vi "Remote Command Sender ver1.vi"() -> ()   [LabVIEW 2016]
panel:
  in  "Max Vacuum":dbl=600.0
  in  "Go 2 Assign Point":bool
  in  "Assign Point":dbl[](array[numeric])=[0.0, 5.0] min=0.5 max=1.5 step=0.05
  out "remote sender engaged":bool
  in  "emergency alarm bit":bool
  in  "Scaling Array":dbl[](array[numeric])=[1.0, 1.0, 1.0] min=0.5 max=1.5 step=0.05
  in  "Rotation Array":dbl[](array[numeric])=[0.0, 0.0, 0.0] min=-30.0 max=30.0 step=1.0
  in  "Translation Array":dbl[](array[numeric])=[0.0, 0.0, 0.0] min=-3.0 max=3.0 step=0.01
  in  "OCT Z-Axis cmd":dbl step=0.5
  in  "stop":bool
  in  "L1":sgl
  in  "L2":sgl
  in  "L3 (L3=20 is RCM)":sgl
  in  "L4":sgl
  in  "gripper":sgl
  in  "down_pedal":sgl format="%.2f"
  in  "up_pedal":bool
  in  "left_pedal":bool
  in  "right_pedal":bool
  in  "StagePosition - X":dbl=6.0
  in  "StagePosition - Y":dbl=6.0
  in  "StagePosition - Z":dbl=6.0
  # "x scaling"
  # "y scaling"
  # "z scaling"
  # "x rotation"
  # "[deg]"
  # "y rotation"
  # "[deg]"
  # "z rotation"
  # "[deg]"
  # "x translation"
  # "[mm]"
  # "y translation"
  # "[mm]"
  # "z translation"
  # "[mm]"
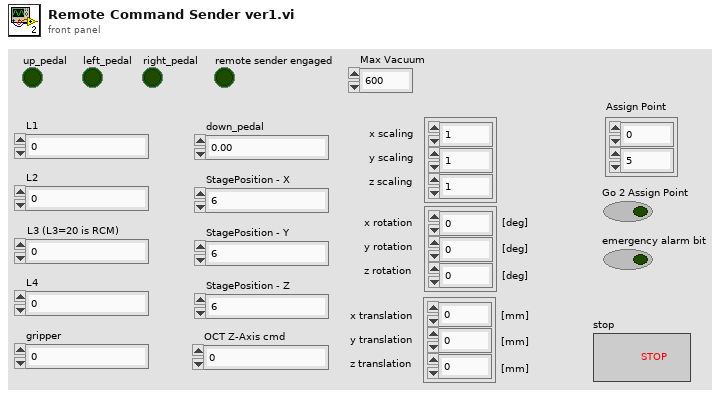
[diagram p1: front panel]
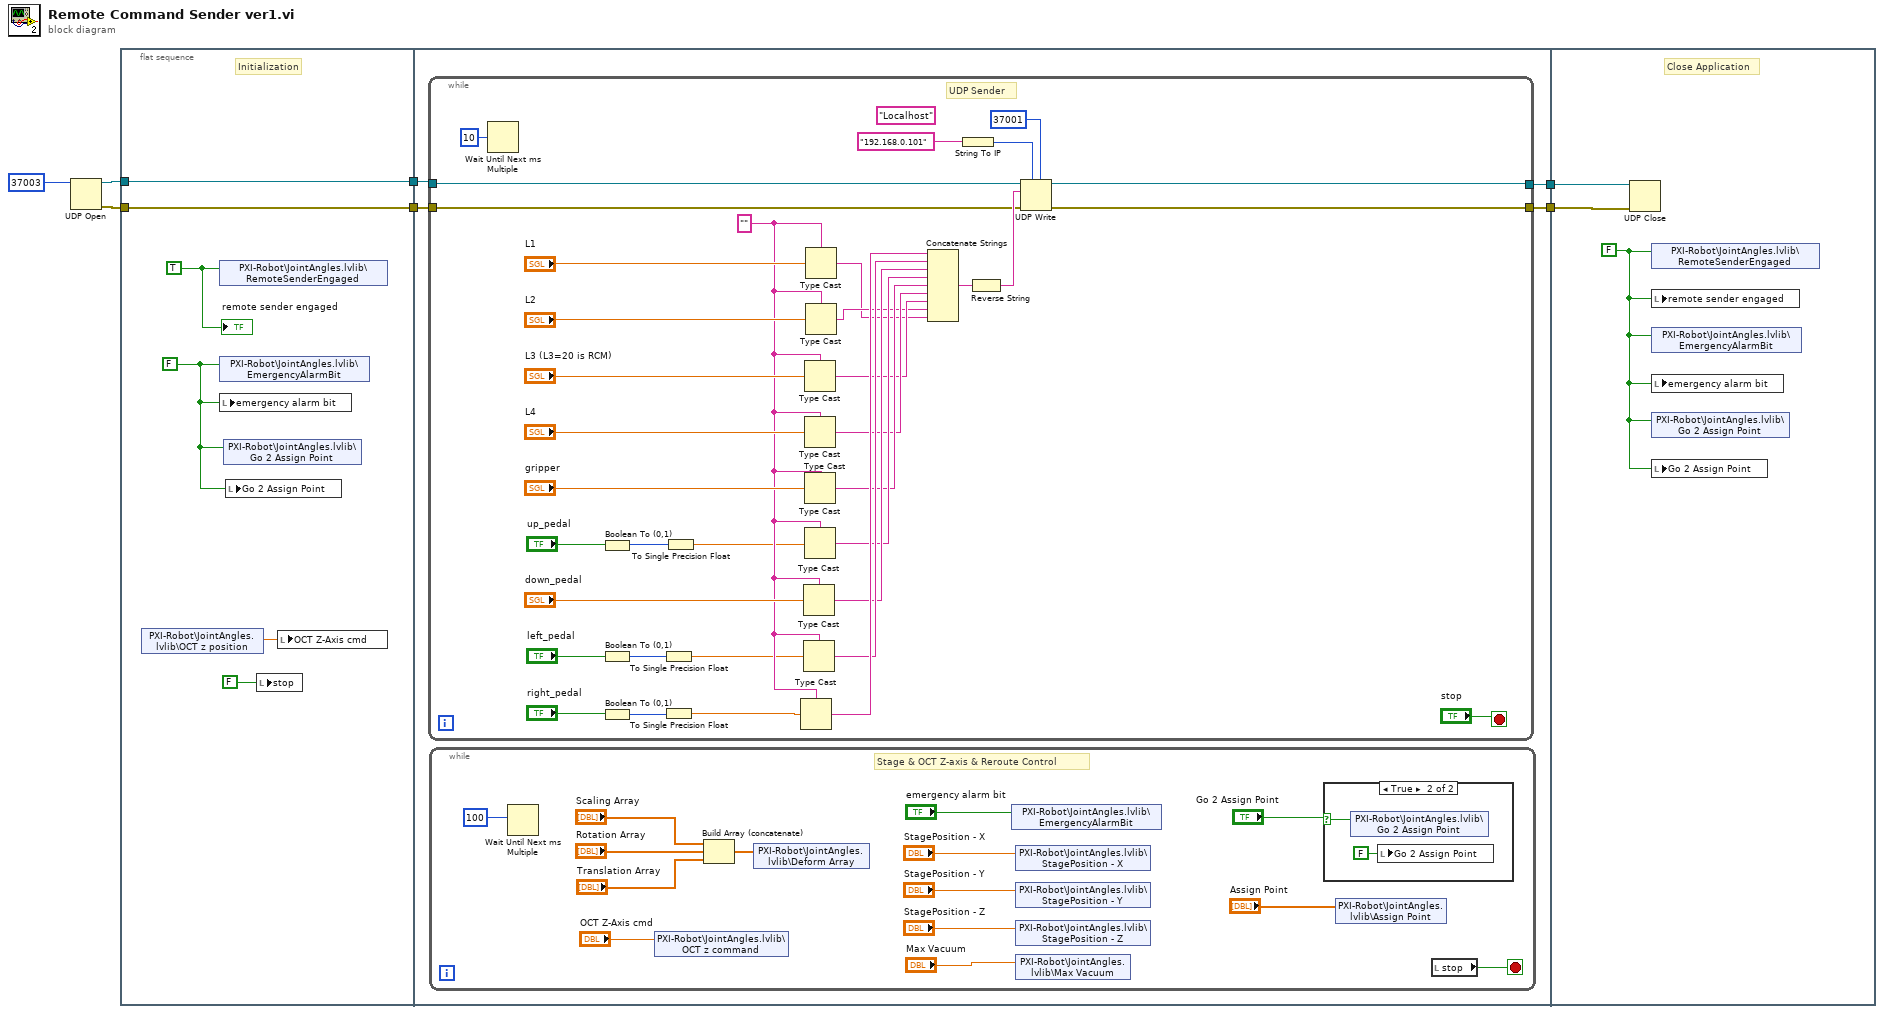
[diagram p0: block diagram]
diagram:
  n1 = UDP Open(11:u16 37003 ("port")) -> (port=w6:refnum<k16>, 0:w5:errorcluster)  [unwired: 4 in, 1 out]
  n2 = flat-sequence {
    tunnel: w5 -> [w12]
    tunnel: w6 -> [w13]
    tunnel: [w13] -> w4
    tunnel: [w12] -> w3
    tunnel: w4 -> [w17]
    tunnel: w3 -> [w16]
    tunnel: [w15] -> w2
    tunnel: [w14] -> w1
    tunnel: w2 -> [w72]
    tunnel: w1 -> [w71]
    frame #0 {
      w8 = FALSE ("EmergencyAlarmBit")
      w10 = TRUE ("RemoteSenderEngaged")
      # "Initialization"
      n3 = shared-variable "PXI-Robot\\JointAngles.lvlib\\OCT z position"() -> (w11:dbl)  [unwired: 1 in, 1 out]
      n4 = shared-variable "PXI-Robot\\JointAngles.lvlib\\RemoteSenderEngaged"(w10) -> ()  [unwired: 1 in, 1 out]
      n5 = shared-variable "PXI-Robot\\JointAngles.lvlib\\EmergencyAlarmBit"(w8) -> ()  [unwired: 1 in, 1 out]
      n6 = local write "emergency alarm bit"(w8) -> ()
      n7 = shared-variable "PXI-Robot\\JointAngles.lvlib\\Go 2 Assign Point"(w8) -> ()  [unwired: 1 in, 1 out]
      n8 = local write "Go 2 Assign Point"(w8) -> ()
      n9 = local write "stop"(FALSE ("stop")) -> ()
      n10 = local write "OCT Z-Axis cmd"(w11) -> ()
      "remote sender engaged" <- w10
    }
    frame #1 {
      n11 = while {
        tunnel: w17 -> [w62]
        tunnel: [w68] -> w15
        tunnel: w16 -> [w61]
        tunnel: [w67] -> w14
        stop <- "stop" stop-if-true
        (unwired) "Localhost" ("reversed")
        w51 = "" ("reversed")
        # "UDP Sender"
        n12 = Wait Until Next ms Multiple(millisecond multiple=u32 10) -> ()  [unwired: 1 out]
        n13 = Boolean To (0,1)(Boolean="up_pedal") -> (0, 1=w41:i16)
        n14 = Boolean To (0,1)(Boolean="left_pedal") -> (0, 1=w37:i16)
        n15 = Boolean To (0,1)(Boolean="right_pedal") -> (0, 1=w39:i16)
        n16 = To Single Precision Float(number=w37) -> (single precision float=w36:sgl)
        n17 = To Single Precision Float(number=w39) -> (single precision float=w38:sgl)
        n18 = To Single Precision Float(number=w41) -> (single precision float=w40:sgl)
        n19 = Type Cast(type=w51, x=w38) -> (*(type *) &x=w50:string)
        n20 = Type Cast(type=w51, x="down_pedal") -> (*(type *) &x=w48:string)
        n21 = Type Cast(type=w51, x=w36) -> (*(type *) &x=w49:string)
        n22 = Type Cast(type=w51, x="L3 (L3=20 is RCM)") -> (*(type *) &x=w44:string)
        n23 = Type Cast(type=w51, x="L4") -> (*(type *) &x=w45:string)
        n24 = Type Cast(type=w51, x="gripper") -> (*(type *) &x=w46:string)
        n25 = Type Cast(type=w51, x=w40) -> (*(type *) &x=w47:string)
        n26 = Type Cast(type=w51, x="L1") -> (*(type *) &x=w42:string)
        n27 = Type Cast(type=w51, x="L2") -> (*(type *) &x=w43:string)
        n28 = Concatenate Strings(w50, w49, w48, w47, w46, w45, w44, w43, w42) -> (w66:string)
        n29 = String To IP(1:"192.168.0.101" ("reversed")) -> (0:w64:u32)
        n30 = Reverse String(1:w66) -> (0:w65:string)
        n31 = UDP Write(address=w64, port or service name=u16 37001, connection ID=w62, data in=w65, 8:w61) -> (error out=w67:errorcluster, 3:w68:refnum<k16>)  [unwired: 1 in]
      }
      n32 = while {
        stop <- w26 stop-if-true
        # "Stage & OCT Z-axis & Reroute Control"
        n33 = Wait Until Next ms Multiple(millisecond multiple=u32 100 ("milliseconds to wait")) -> ()  [unwired: 1 out]
        n34 = shared-variable "PXI-Robot\\JointAngles.lvlib\\OCT z command"("OCT Z-Axis cmd") -> ()  [unwired: 1 in, 1 out]
        n35 = Build Array (concatenate)("Scaling Array", "Rotation Array", "Translation Array") -> (w28:dbl[])
        n36 = shared-variable "PXI-Robot\\JointAngles.lvlib\\Deform Array"(w28) -> ()  [unwired: 1 in, 1 out]
        n37 = shared-variable "PXI-Robot\\JointAngles.lvlib\\EmergencyAlarmBit"("emergency alarm bit") -> ()  [unwired: 1 in, 1 out]
        n38 = shared-variable "PXI-Robot\\JointAngles.lvlib\\StagePosition - X"("StagePosition - X") -> ()  [unwired: 1 in, 1 out]
        n39 = shared-variable "PXI-Robot\\JointAngles.lvlib\\StagePosition - Y"("StagePosition - Y") -> ()  [unwired: 1 in, 1 out]
        n40 = shared-variable "PXI-Robot\\JointAngles.lvlib\\StagePosition - Z"("StagePosition - Z") -> ()  [unwired: 1 in, 1 out]
        n41 = shared-variable "PXI-Robot\\JointAngles.lvlib\\Max Vacuum"("Max Vacuum") -> ()  [unwired: 1 in, 1 out]
        n42 = case shown="True" "Go 2 Assign Point" {
          selector: "Go 2 Assign Point" -> [_ w33]
          frame False {
          }
          frame True {
            n43 = shared-variable "PXI-Robot\\JointAngles.lvlib\\Go 2 Assign Point"(w33) -> ()  [unwired: 1 in, 1 out]
            n44 = local write "Go 2 Assign Point"(FALSE ("Go 2 Assign Point")) -> ()
          }
        }
        n45 = shared-variable "PXI-Robot\\JointAngles.lvlib\\Assign Point"("Assign Point") -> ()  [unwired: 1 in, 1 out]
        n46 = local read "stop"() -> (w26:bool)
      }
    }
    frame #2 {
      w70 = FALSE ("RemoteSenderEngaged")
      # "Close Application"
      n47 = UDP Close(connection ID=w72, 8:w71) -> ()  [unwired: 2 out]
      n48 = shared-variable "PXI-Robot\\JointAngles.lvlib\\RemoteSenderEngaged"(w70) -> ()  [unwired: 1 in, 1 out]
      n49 = local write "remote sender engaged"(w70) -> ()
      n50 = shared-variable "PXI-Robot\\JointAngles.lvlib\\EmergencyAlarmBit"(w70) -> ()  [unwired: 1 in, 1 out]
      n51 = local write "emergency alarm bit"(w70) -> ()
      n52 = shared-variable "PXI-Robot\\JointAngles.lvlib\\Go 2 Assign Point"(w70) -> ()  [unwired: 1 in, 1 out]
      n53 = local write "Go 2 Assign Point"(w70) -> ()
    }
  }
